vi "Set Personality.vi"(0 "GEA2 Reference In":refnum<k24>, 5 "Personality":u8, 11 "Error In":errorcluster) -> (4 "GEA2 Reference Out":refnum<k24>, 6 "Pass/Fail?":bool=TRUE, 8 "Report Text":string, 15 "Error Out":errorcluster)   [LabVIEW 2018, in "TLMB.lvlib"]
doc: "Use this VI to set the washer personality."
uses:
  Projects/TLMB.lvlib
  D:/Common/LabVIEW GEA2 Toolkit/source/GEA3 DLL Source/GeaCommunication.dll
  Common/LabVIEW GEA2 Toolkit/source/GEA3 DLL Source/GeaCommunication.dll
  Common/LabVIEW GEA2 Toolkit/GEA3/type defs/Source_Destination.ctl
  Common/LabVIEW GEA2 Toolkit/GEA3/type defs/ERD Read Data In.ctl
  Common/LabVIEW GEA2 Toolkit/GEA3/type defs/Data Type.ctl
  Common/LabVIEW GEA2 Toolkit/GEA3/type defs/ERD Write Data In.ctl
  C:/Users/iallatyp/Desktop/New folder/GEA3/library/GEA2_Toolkit.lvlib
panel:
  in  "Standalone?":bool
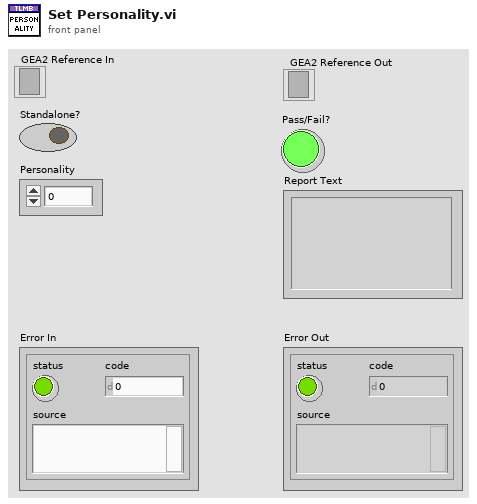
[diagram p1: front panel]
types:
  T1 = typedef "GEA2_Toolkit.lvlib/ERD Read Data In.ctl" = cluster{"ERD Number":u16, "Data Type":T2}
  T2 = typedef "GEA2_Toolkit.lvlib/Data Type.ctl" = enum16{"string", "boolean", "uint8_t", "uint16_t", "uint32_t", "uint64_t", "int8_t", "int16_t", "int32_t", "int64_t"}
  T3 = typedef "GEA2_Toolkit.lvlib/Source_Destination.ctl" = cluster{"Source":u8, "Destination":u8}
  T4 = typedef "GEA2_Toolkit.lvlib/ERD Read Data Out.ctl" = cluster{"ERD Number":u16, "Data":string}
  T5 = typedef "GEA2_Toolkit.lvlib/ERD Write Data In.ctl" = cluster{"ERD Number":u16, "Data Type":T2, "Data":string}
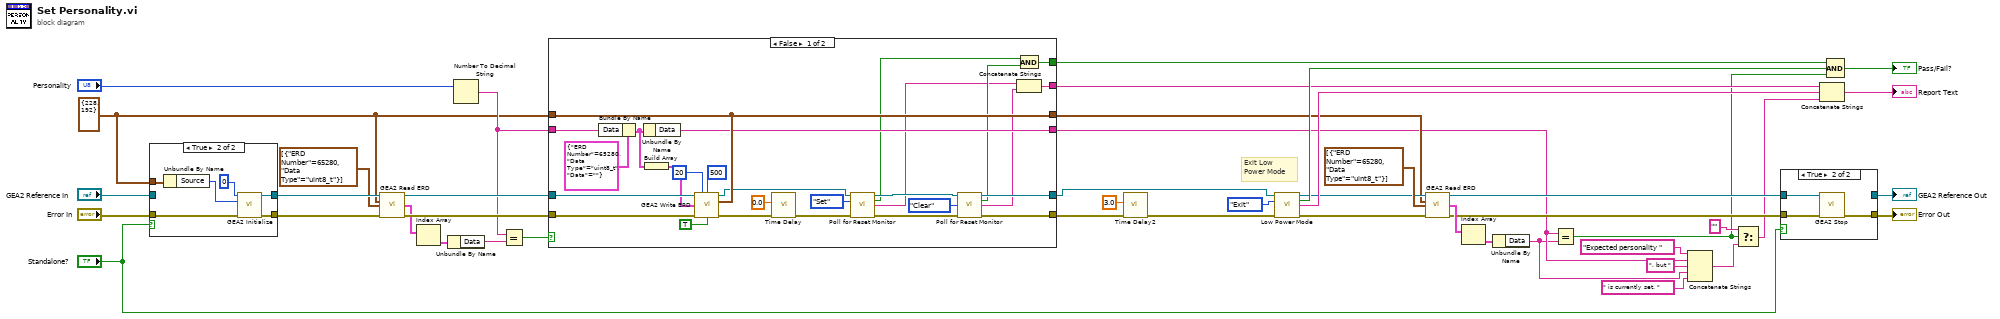
[diagram p0: block diagram]
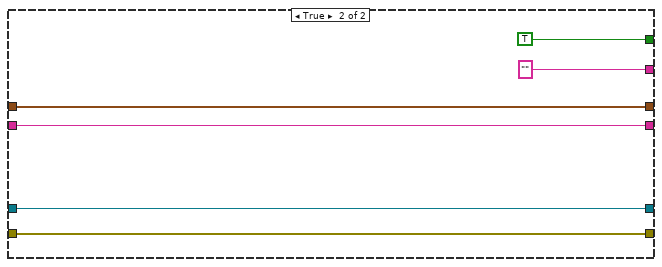
[diagram p2: hidden frame]
diagram:
  w23 = T3 {"Source"=228, "Destination"=192} ("GEA Inputs")
  # "Exit Low \nPower Mode"
  n1 = case shown="True" "Standalone?" {
    tunnel: "Error In" -> [w46 w53]
    tunnel: [w46 w52] -> w32
    tunnel: "GEA2 Reference In" -> [w47 _]
    tunnel: [w47 w51] -> w33
    tunnel: w23 -> [_ w49]
    frame False {
    }
    frame True {
      n2 = Unbundle By Name(w49) -> ("Source"=w50:u8)
      n3 = call "GEA2 Initialize.vi"("Board Index"=0, "Source Address"=w50, "error in"=w53) -> ("GEA2 Reference Out"=w51:refnum<k24>, "error out"=w52:errorcluster)  [unwired: 10 in, 1 out]
    }
  }
  n4 = call "GEA2 Read ERD.vi"("GEA2 Reference In"=w33, "GEA Inputs"=w23, "Read ERD List"=T1[] [{"ERD Number"=65280, "Data Type"=enum."uint8_t"}], "Error In"=w32) -> ("GEA2 Reference Out"=w31:refnum<k24>, "ERD Data Out"=w29:T4[], "Error Out"=w30:errorcluster)  [unwired: 8 in, 1 out]
  n5 = Index Array(array=w29) -> (element=w28:T4)  [unwired: 1 in]
  n6 = Unbundle By Name(w28) -> ("Data"=w26:string)
  n7 = Number To Decimal String(number="Personality") -> (decimal integer string=w24:string)  [unwired: 1 in]
  n8 = Equal?(x=w24, y=w26) -> (x = y?=w25:bool)
  n9 = case shown="False" w25 {
    tunnel: [w63 w85] -> w2
    tunnel: [w58 w86] -> w38
    tunnel: w31 -> [w79 w86]
    tunnel: w30 -> [w78 w85]
    tunnel: w24 -> [w75 w81]
    tunnel: w23 -> [w72 w82]
    tunnel: [w74 TRUE] -> w22
    tunnel: [w73 ""] -> w21
    tunnel: [w72 w82] -> w13
    tunnel: [w70 w81] -> w7
    frame False {
      n10 = Bundle By Name(cluster=T5 {"ERD Number"=65280, "Data Type"=enum."uint8_t", "Data"=""} ("ERD Write Data In"), "Data"=w75) -> (w71:T5)
      n11 = Unbundle By Name(w71) -> ("Data"=w70:string)
      n12 = Build Array(w71) -> (w76:T5[])
      n13 = call "GEA2 Write ERD.vi"("GEA2 Reference In"=w79, "# of Tries"=20 ("Retry Count"), "Read Timeout (ms)"=u32 500, "GEA Inputs"=w72, "Write ERD List"=w76, "Error In"=w78, "Verify ERD Response?"=TRUE) -> ("GEA2 Reference Out"=w60:refnum<k24>, "Error Out"=w80:errorcluster)  [unwired: 6 in, 1 out]
      n14 = call "Time Delay"("error in (no error)"=w80, "Delay Time (s)"=0.0) -> ("error out"=w65:errorcluster)  [unwired: 9 in]
      n15 = call "Poll for Reset Monitor.vi"("GEA2 Reference In"=w60, "Status"=enum16{"Clear", "Set"}."Set", "Error In"=w65) -> ("GEA2 Reference Out"=w59:refnum<k24>, "Pass/Fail?"=w57:bool, "Report Text"=w55:string, "Error Out"=w64:errorcluster)  [unwired: 8 in, 1 out]
      n16 = call "Poll for Reset Monitor.vi"("GEA2 Reference In"=w59, "Status"=enum16{"Clear", "Set"}."Clear", "Error In"=w64) -> ("GEA2 Reference Out"=w58:refnum<k24>, "Pass/Fail?"=w56:bool, "Report Text"=w54:string, "Error Out"=w63:errorcluster)  [unwired: 8 in, 1 out]
      n17 = Concatenate Strings(w55, w54) -> (w73:string)
      n18 = Compound Arithmetic op=AND(w57, w56) -> (w74:bool)
    }
    frame True {
    }
  }
  n19 = call "Time Delay2"("error in (no error)"=w2, "Delay Time (s)"=3.0) -> ("error out"=w1:errorcluster)  [unwired: 9 in]
  n20 = call "Low Power Mode.vi"("GEA2 Reference In"=w38, "Action"=enum16{"Enter", "Exit"}."Exit", "Error In"=w1) -> ("GEA2 Reference Out"=w17:refnum<k24>, "Pass/Fail?"=w36:bool, "Report Text"=w40:string, "Error Out"=w16:errorcluster)  [unwired: 9 in]
  n21 = call "GEA2 Read ERD.vi"("GEA2 Reference In"=w17, "GEA Inputs"=w13, "Read ERD List"=T1[] [{"ERD Number"=65280, "Data Type"=enum."uint8_t"}], "Error In"=w16) -> ("GEA2 Reference Out"=w14:refnum<k24>, "ERD Data Out"=w18:T4[], "Error Out"=w15:errorcluster)  [unwired: 8 in, 1 out]
  n22 = Index Array(array=w18) -> (element=w19:T4)  [unwired: 1 in]
  n23 = Unbundle By Name(w19) -> ("Data"=w5:string)
  n24 = Equal?(x=w7, y=w5) -> (x = y?=w11:bool)
  n25 = Concatenate Strings("Expected personality " ("string"), w7, ", but " ("string"), w5, " is currently set. " ("string")) -> (w8:string)
  n26 = Select(t="" ("Report Text"), s=w11, f=w8) -> (s? t:f=w10:string)
  n27 = case shown="True" "Standalone?" {
    tunnel: w15 -> [w88 w91]
    tunnel: [w88 w90] -> w45
    tunnel: [w87 _] -> w44
    tunnel: w14 -> [w87 w89]
    frame False {
    }
    frame True {
      n28 = call "GEA2 Stop.vi"("GEA2 Reference In"=w89, "Error In"=w91) -> ("Error Out"=w90:errorcluster)  [unwired: 13 in]
    }
  }
  "Error Out" <- w45
  "GEA2 Reference Out" <- w44
  n29 = Concatenate Strings(w21, w40, w10) -> (→"Report Text":string)
  n30 = Compound Arithmetic op=AND(w22, w36, w11) -> (→"Pass/Fail?":bool)
